vi "Shooter_Turret_Motor.vi"(0 "MotorControlDevRef":T2={"DeviceStatus"={"status"=FALSE, "code"=0, "source"=""}, "Type"=enum."PWM", "PWM"={"PWM Channel"=enum."Invalid", "DeadBand"={"Name"="", "maxPositivePwm"=0, "minPositivePwm"=0, "centerPwm"=0, "maxNegativePwm"=0, "minNegativePwm"=0, "angularRange"=0}}, "CAN"={"Device Number"=0, "SetOutput VI Ref"=variant(refnum<vi> refnum), "GetOutput VI Ref"=variant(refnum<vi> refnum), "Enable VI Ref"=variant(refnum<vi> refnum), "Disable VI Ref"=variant(refnum<vi> refnum), "Data"=variant}, "Invert"=FALSE}, 1 "Dt_ Input":dbl, 2 "Pot_Input":dbl, 3 "Pot_Wanted_Value":dbl, 4 "Turret_Clockwise?":bool, 5 "Turret_Counterclockwise?":bool, 6 "Invert?":bool, 7 "PID gains":T1={"proportional gain (Kc)"=1.0, "integral time (Ti, min)"=0.01, "derivative time (Td, min)"=0.0} {"derivative time (Td, min)" format="%.3f"; "integral time (Ti, min)" format="%.3f"; "proportional gain (Kc)" format="%.3f"}) -> (20 "Dt_Output":dbl)   [LabVIEW 2016]
uses:
  <vilib>/Rock Robotics/WPI/MotorControl/WPI_MotorControlDeviceRef.ctl
  <vilib>/Rock Robotics/WPI/MotorControl/WPI_MotorControlType.ctl
  <vilib>/Rock Robotics/SystemInterfaces/DIO/FPGA_DIOPWMChannel.ctl
  <vilib>/Rock Robotics/WPI/PWM/WPI_PWMDeadband.ctl
  <vilib>/addons/control/pid/pid.llb/PID (DBL).vi
  <vilib>/addons/control/pid/NI_PID_pid.lvlib
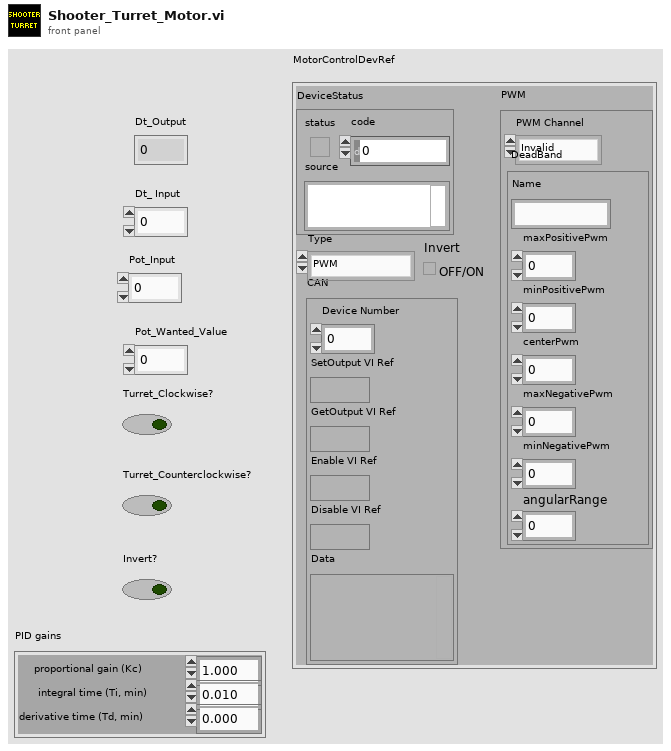
[diagram p1: front panel]
types:
  T1 = cluster{"proportional gain (Kc)":dbl, "integral time (Ti, min)":dbl, "derivative time (Td, min)":dbl}
  T2 = typedef "WPI_MotorControlDeviceRef.ctl" = cluster{"DeviceStatus":errorcluster, "Type":T3, "PWM":cluster{"PWM Channel":T4, "DeadBand":T5}, "CAN":cluster{"Device Number":u8, "SetOutput VI Ref":variant, "GetOutput VI Ref":variant, "Enable VI Ref":variant, "Disable VI Ref":variant, "Data":variant}, "Invert":bool}
  T3 = typedef "WPI_MotorControlType.ctl" = enum16{"PWM", "CAN"}
  T4 = typedef "FPGA_DIOPWMChannel.ctl" = enum8{"PWM 0", "PWM 1", "PWM 2", "PWM 3", "PWM 4", "PWM 5", "PWM 6", "PWM 7", "PWM 8", "PWM 9", "PWM MXP 0", "PWM MXP 1", "PWM MXP 2", "PWM MXP 3", "PWM MXP 4", "PWM MXP 5", "PWM MXP 6", "PWM MXP 7", "PWM MXP 8", "PWM MXP 9", "Invalid"}
  T5 = typedef "WPI_PWMDeadband.ctl" = cluster{"Name":string, "maxPositivePwm":i32, "minPositivePwm":i32, "centerPwm":i32, "maxNegativePwm":i32, "minNegativePwm":i32, "angularRange":u16}
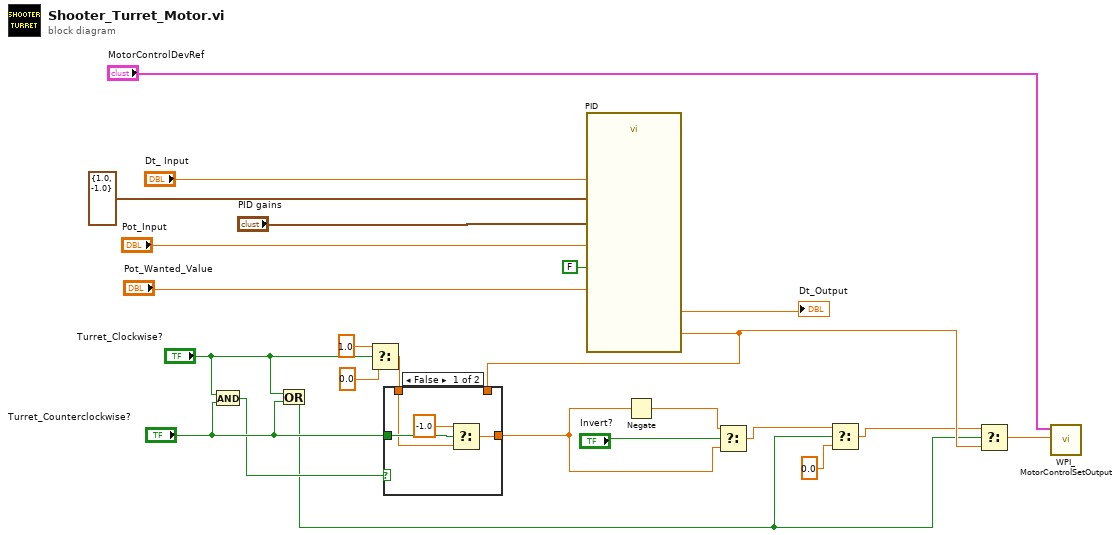
[diagram p0: block diagram]
diagram:
  n1 = And(x="Turret_Clockwise?", y="Turret_Counterclockwise?") -> (x .and. y?=w3:bool)
  n2 = Or(x="Turret_Clockwise?", y="Turret_Counterclockwise?") -> (x .or. y?=w2:bool)
  n3 = Select(t=1.0, s="Turret_Clockwise?", f=0.0) -> (s? t:f=w20:dbl)
  n4 = call-poly <vilib>:"PID.vi"("reinitialize? (F)"=FALSE, "output range"=cluster{"output high":dbl, "output low":dbl} {"output high"=1.0, "output low"=-1.0}, "dt (s)"="Dt_ Input", "PID gains"="PID gains", "process variable"="Pot_Input", "setpoint"="Pot_Wanted_Value") -> ("dt out (s)"=→"Dt_Output":dbl, "output"=w6:dbl)  [unwired: 4 in]
  n5 = case shown="False" w3 {
    tunnel: "Turret_Counterclockwise?" -> [w27 _]
    tunnel: w20 -> [w26 _]
    tunnel: [w24 w28] -> w18
    tunnel: w6 -> [_ w28]
    frame False {
      n6 = Select(t=-1.0, s=w27, f=w26) -> (s? t:f=w24:dbl)
    }
    frame True {
    }
  }
  n7 = Negate(x=w18) -> (-x=w17:dbl)
  n8 = Select(t=w17, s="Invert?", f=w18) -> (s? t:f=w5:dbl)
  n9 = Select(t=w5, s=w2, f=0.0) -> (s? t:f=w1:dbl)
  n10 = Select(t=w1, s=w2, f=w6) -> (s? t:f=w9:dbl)
  n11 = call <vilib>:"WPI_MotorControlSetOutput.vi"("Output"=w9, "MotorControlDevRef"="MotorControlDevRef") -> ()  [unwired: 7 in, 3 out]
